vi "VI Stopped FGV.vi"() -> ()   [LabVIEW 2012]
doc: "SciScan 1.2 160622"
panel:
  in  "VI Name (for Get State)":string
  in  "Action":enum16{"Set Stopped Status", "Get Status List"}(ring)
  out "Error Out":errorcluster
  in  "Error In":errorcluster
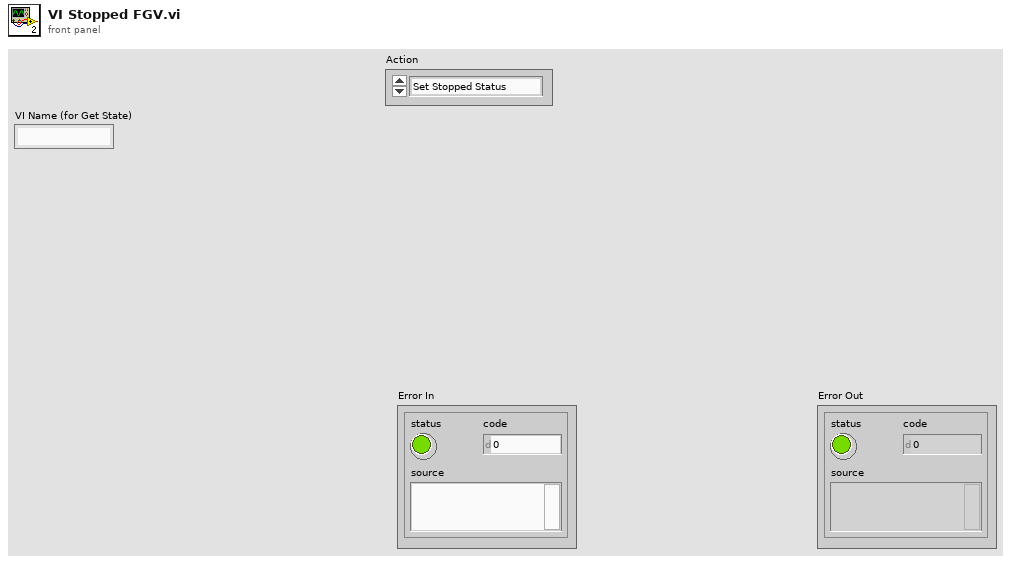
[diagram p1: front panel]
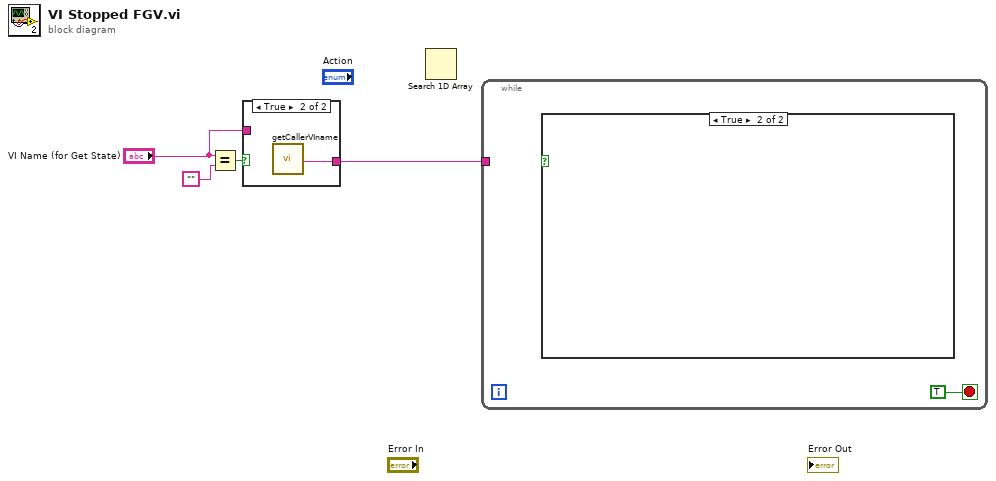
[diagram p0: block diagram]
diagram:
  n1 = Equal?(x="VI Name (for Get State)", y="") -> (x = y?=w3:bool)
  n2 = case shown="True" w3 {
    tunnel: [w5 w6] -> w1
    tunnel: "VI Name (for Get State)" -> [w5 _]
    frame False {
    }
    frame True {
      n3 = call "getCallerVIname.vi"() -> ("VI name"=w6:string)  [unwired: 19 in]
    }
  }
  n4 = Search 1D Array() -> ()  [unwired: 3 in, 1 out]
  n5 = while {
    tunnel: w1 -> [_]
    stop <- TRUE stop-if-true
    n6 = case shown="True" {
      selector: _ -> [_ _]
      frame False {
      }
      frame True {
      }
    }
  }
